vi "Pressure_control_April2018.vi"(7 "Run Sequence":bool, 8 "user sequence, present (s) in, current step in, seq time in":T7, 9 "pressure parameters in":T4={"valve % open"=100.0, "Desired pressure"=0.0, "set Vapor sccm"=0.0, "set Gas sccm"=0.0, "Valve mode"=enum."% Open", "Pressure Mode"=enum."Abs. pressure", "analyte partial pressure"=100.0} caption="Set pressure parameters" {"analyte partial pressure" min=0.0 max=100.0 step=5.0; "set Gas sccm" min=0 max=200 step=5; "set Vapor sccm" min=0 max=200 step=5; "Desired pressure" min=0.0 max=760.0 step=5.0; "valve % open" min=0.0 max=100.0 step=5.0 format="%#_2f"}, 11 "pressure control on?/daq IDs/errors":T3) -> (0 "current step # out, shift register time out, seq button on?":T6, 1 "sequence over? USE THIS TO REINITIALIZE RUN SEQUENCE BUTTON SO PROGRAM ENDS":bool, 2 "save press/RH/gasflow/vaporflow - read valve position/pressure/vaporflow/gasflow":T5, 3 "pressure control on?/daq IDs/errors out":T2, 4 "sequence end date/time string":string, 5 "abs_t, delta_t, abs_p, delta_p":T1)   [LabVIEW 2014]
uses:
  <vilib>/DAQmx/read.llb/DAQmx Read (Analog 1D DBL NChan 1Samp).vi
  <vilib>/DAQmx/write.llb/DAQmx Write (Analog 1D DBL NChan 1Samp).vi
panel:
  # "100%"
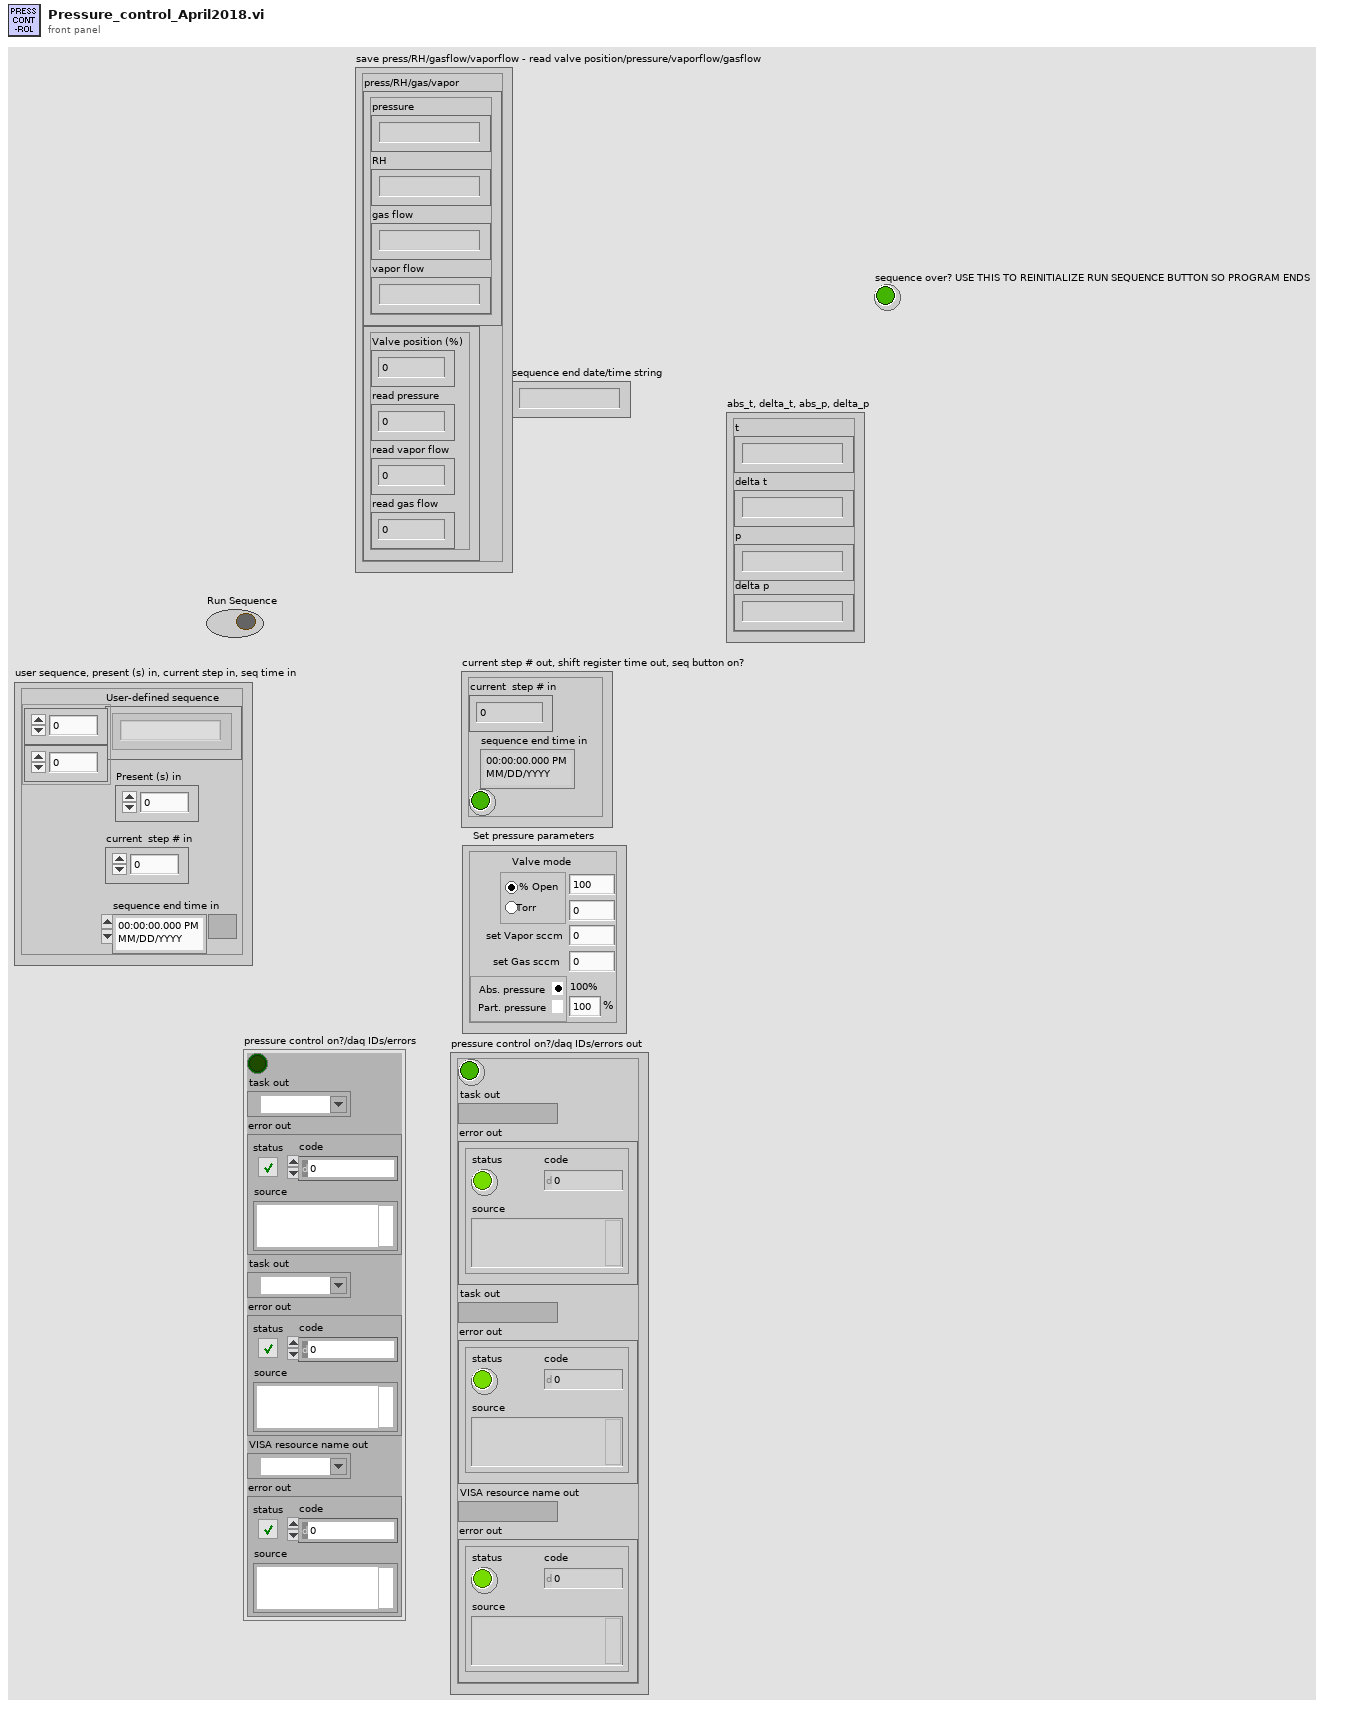
[diagram p1: front panel]
types:
  T1 = cluster{"t":string, "delta t":string, "p":string, "delta p":string}
  T2 = cluster{"Boolean":bool, "task out":refnum<k21>, "error out":errorcluster, "task out":refnum<k21>, "error out":errorcluster, "VISA resource name out":refnum<visa-resource-name>, "error out":errorcluster}
  T3 = cluster{bool, "task out":refnum<k21>, "error out":errorcluster, "task out":refnum<k21>, "error out":errorcluster, "VISA resource name out":refnum<visa-resource-name>, "error out":errorcluster}
  T4 = cluster{"valve % open":dbl, "Desired pressure":dbl, "set Vapor sccm":sgl, "set Gas sccm":sgl, "Valve mode":enum32{"% Open", "Torr "}, "Pressure Mode":enum32{"Abs. pressure", " Part. pressure"}, "analyte partial pressure":dbl}
  T5 = cluster{"press/RH/gas/vapor":cluster{"pressure":string, "RH":string, "gas flow":string, "vapor flow":string}, "Cluster":cluster{"Valve position (%)":dbl, "read pressure":dbl, "read vapor flow":dbl, "read gas flow":dbl}}
  T6 = cluster{"current  step # in":i32, "sequence end time in":timestamp, "Boolean":bool}
  T7 = cluster{"User-defined sequence":string[][], "Present (s) in":dbl, "current  step # in":i32, "sequence end time in":timestamp}
  T8 = cluster{"Elapsed Time (s)":string, "Elapsed Time (s)":string, "String":string, string}
  T9 = cluster{"Valve position (%)":dbl, "pressure":dbl, "vapor flow":dbl, "gas flow":dbl}
  T10 = cluster{"pressure":string, "RH":string, "gas flow":string, "vapor flow":string}
  T11 = cluster{"String":dbl, "String":dbl, "Pressure Control":u32}
  T12 = cluster{"Valve position (%)":dbl, "read pressure":dbl, "read vapor flow":dbl, "read gas flow":dbl}
  T13 = cluster{"Elapsed Time (s)":dbl, "Elapsed Time (s)":dbl, "String":dbl, dbl}
  T14 = cluster{bool, "task out":refnum<k21>, "error out":errorcluster, "task out":refnum<k21>, "error out":errorcluster, "VISA Refnum out":refnum<visa-resource-name>, "error out":errorcluster}
  T15 = cluster{"press/RH/gas/vapor":cluster{"pressure":string, "RH":string, "gas flow":string, "vapor flow":string}, cluster{"Valve position (%)":dbl, "read pressure":dbl, "read vapor flow":dbl, "read gas flow":dbl}}
  T16 = cluster{"current  step # in":i32, "sequence end time in":timestamp, bool}
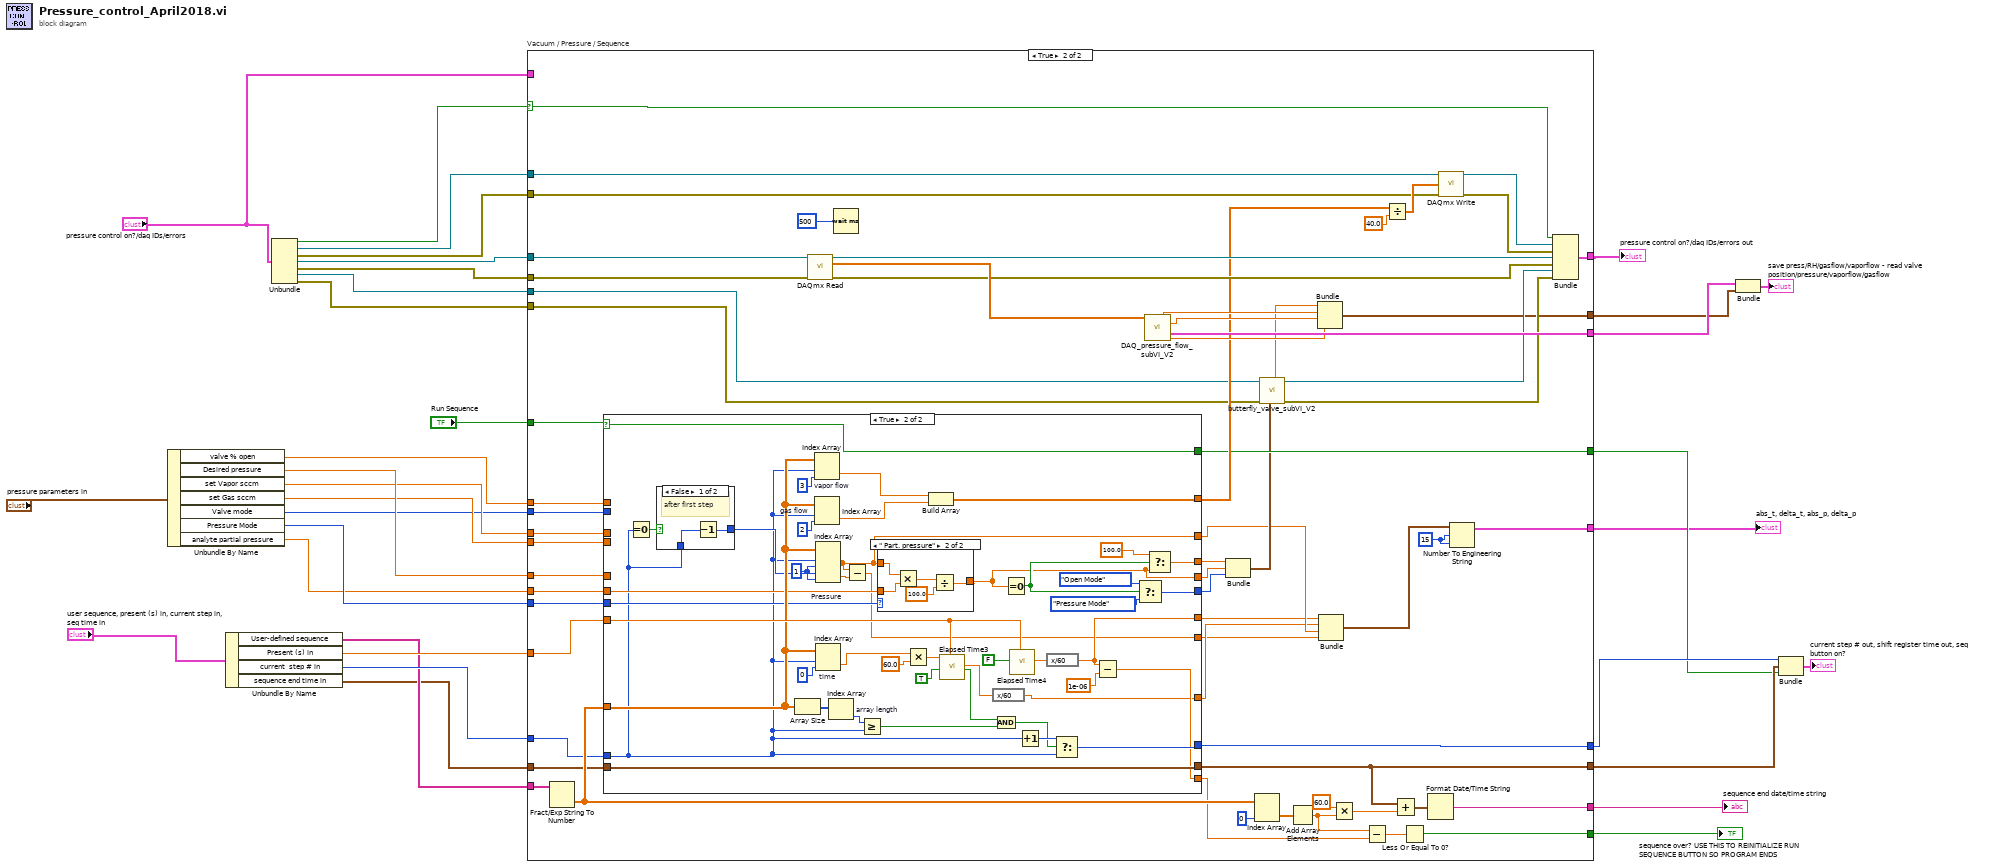
[diagram p0: block diagram]
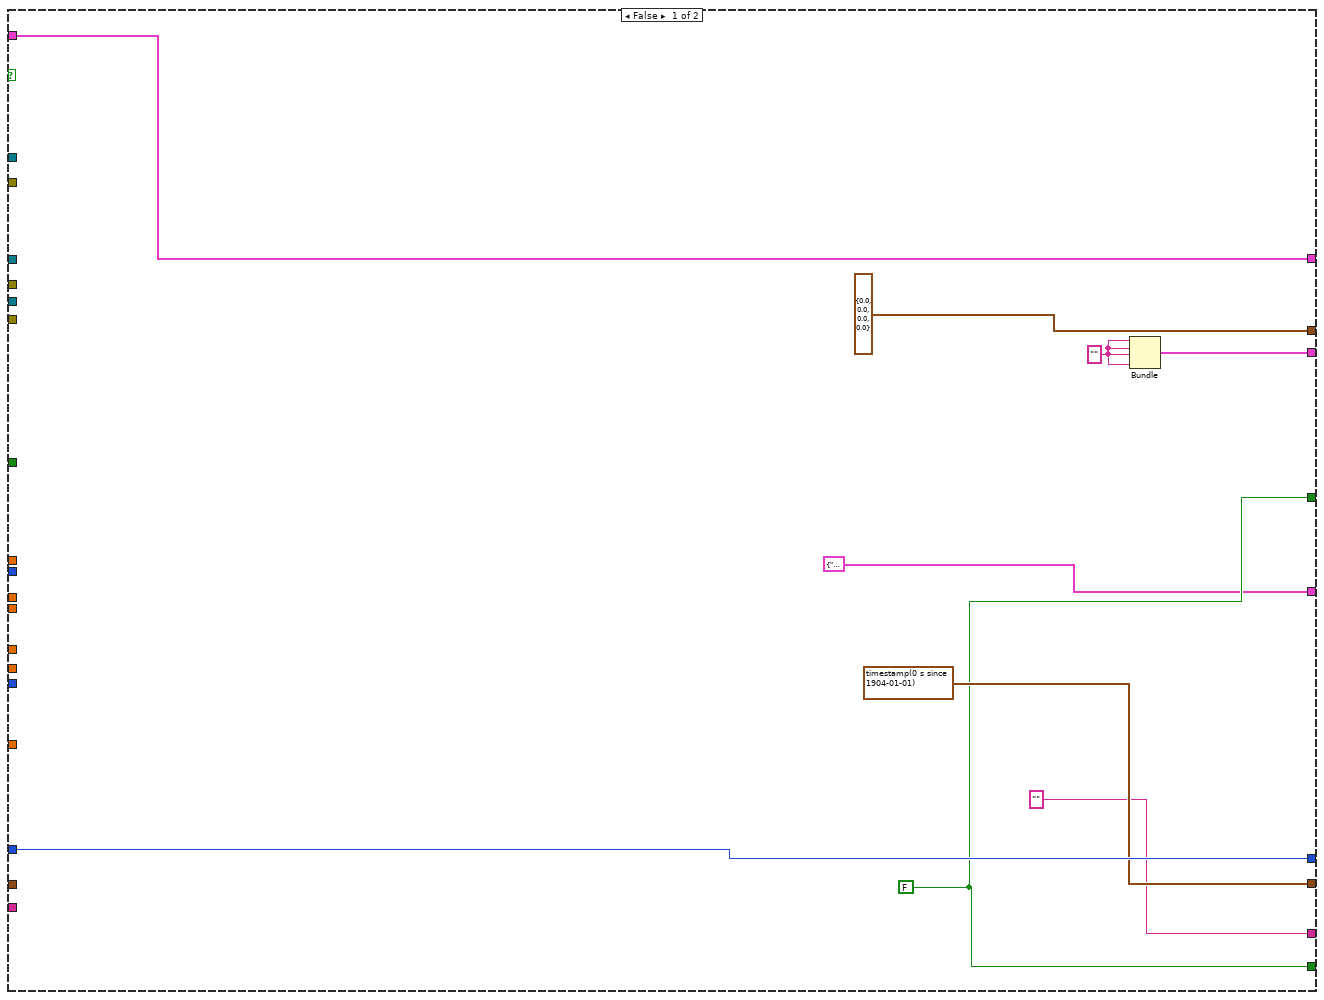
[diagram p2: hidden frame]
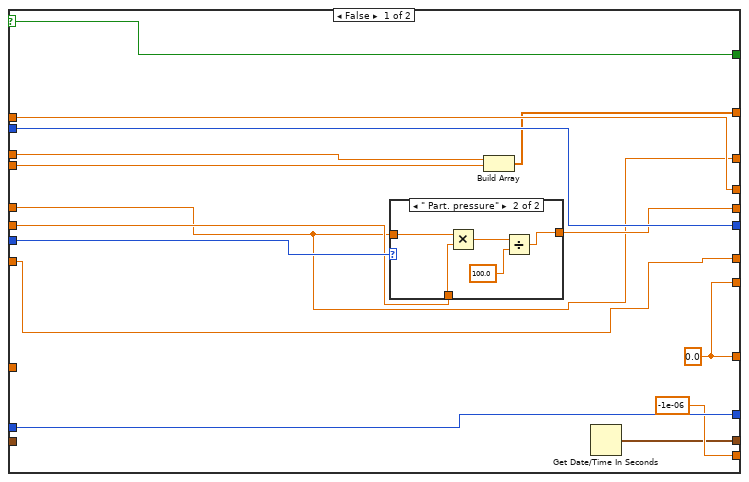
[diagram p3: hidden frame]
diagram:
  n1 = Unbundle By Name("pressure parameters in") -> ("valve % open"=w11:dbl, "Desired pressure"=w15:dbl, "set Vapor sccm"=w13:sgl, "set Gas sccm"=w14:sgl, "Valve mode"=w12:enum32{"% Open", "Torr "}, "Pressure Mode"=w17:enum32{"Abs. pressure", " Part. pressure"}, "analyte partial pressure"=w16:dbl)
  n2 = Unbundle By Name("user sequence, present (s) in, current step in, seq time in") -> ("User-defined sequence"=w27:string[][], "Present (s) in"=w28:dbl, "current  step # in"=w29:i32, "sequence end time in"=w26:timestamp)
  n3 = Unbundle("pressure control on?/daq IDs/errors") -> (w10:bool, "task out"=w9:refnum<k21>, "error out"=w8:errorcluster, "task out"=w7:refnum<k21>, "error out"=w6:errorcluster, "VISA resource name out"=w5:refnum<visa-resource-name>, "error out"=w4:errorcluster)
  n4 = case "Vacuum / Pressure / Sequence" shown="True" w10 {
    selector: w10 -> [_ w50]
    tunnel: w29 -> [w42 w79]
    tunnel: [w42 w59] -> w25
    tunnel: [w37 w77] -> w23
    tunnel: [timestamp(0 s since 1904-01-01) ("seconds since 1Jan1904") w76] -> w24
    tunnel: [w40 w93] -> w21
    tunnel: w27 -> [_ w84]
    tunnel: ["" ("date/time string") w83] -> w33
    tunnel: [T9 {"Valve position (%)"=0.0, "pressure"=0.0, "vapor flow"=0.0, "gas flow"=0.0} w82] -> w20
    tunnel: w28 -> [_ w74]
    tunnel: "Run Sequence" -> [_ w73]
    tunnel: w26 -> [_ w72]
    tunnel: [w37 w71] -> w31
    tunnel: w15 -> [_ w70]
    tunnel: w11 -> [_ w69]
    tunnel: w13 -> [_ w68]
    tunnel: w17 -> [_ w67]
    tunnel: w12 -> [_ w66]
    tunnel: w14 -> [_ w65]
    tunnel: w16 -> [_ w64]
    tunnel: w9 -> [_ w57]
    tunnel: w8 -> [_ w56]
    tunnel: w7 -> [_ w55]
    tunnel: w6 -> [_ w54]
    tunnel: w5 -> [_ w53]
    tunnel: w4 -> [_ w52]
    tunnel: "pressure control on?/daq IDs/errors" -> [w35 _]
    tunnel: [w35 w51] -> w2
    tunnel: [T8 {"Elapsed Time (s)"="", "Elapsed Time (s)"="", "String"="", ""} w45] -> w1
    frame False {
      w37 = FALSE
      w39 = ""
      n5 = Bundle(w39, w39, w39, w39) -> (w40:cluster{string, string, string, string})  [unwired: 1 in]
    }
    frame True {
      w43 = i16 15 ("precision (6)")
      n6 = Fract/Exp String To Number ("user sequence")(string=w84) -> (number=w80:dbl[][])  [unwired: 3 in, 1 out]
      n7 = case "Sequence" shown="True" w73 {
        selector: w73 -> [w116 w154]
        tunnel: w74 -> [w106 w159]
        tunnel: [w119 w160] -> w59
        tunnel: w79 -> [w119 w126]
        tunnel: w65 -> [w114 _]
        tunnel: [w111 w137] -> w63
        tunnel: w80 -> [_ w156]
        tunnel: w66 -> [w118 _]
        tunnel: [w118 w140] -> w62
        tunnel: [-1e-06 w138] -> w75
        tunnel: [w116 w154] -> w77
        tunnel: [w115 w144] -> w58
        tunnel: w69 -> [w115 _]
        tunnel: [w113 w150] -> w78
        tunnel: [w112 w149] -> w76
        tunnel: w72 -> [_ w149]
        tunnel: w70 -> [w107 _]
        tunnel: w64 -> [w108 w148]
        tunnel: w67 -> [w110 w146]
        tunnel: w68 -> [w109 _]
        tunnel: [w107 w128] -> w49
        tunnel: [w106 w135] -> w48
        tunnel: [w105 w133] -> w47
        tunnel: [w105 w127] -> w44
        frame False {
          w105 = 0.0
          n8 = case shown="\" Part. pressure\"" w110 {
            tunnel: [w120 w121] -> w111
            tunnel: w107 -> [w120 w123]
            tunnel: w108 -> [_ w122]
            frame "Abs. pressure", Default {
            }
            frame " Part. pressure" {
              n9 = Multiply(x=w123, y=w122) -> (x*y=w125:dbl)
              n10 = Divide(x=w125, y=100.0 ("Analyte part. press. (%)")) -> (x/y=w121:dbl)
            }
          }
          n11 = Build Array(w109, w114) -> (w113:sgl[])
          n12 = Get Date/Time In Seconds() -> (seconds since 1Jan1904=w112:timestamp)
        }
        frame True {
          w131 = 1 ("disabled index (col)")
          n13 = Equal To 0?(x=w126) -> (x = 0?=w132:bool)
          n14 = case shown="False" w132 {
            tunnel: w126 -> [w171 w172]
            tunnel: [w170 w172] -> w130
            frame False {
              # "after first step"
              n15 = Decrement(x=w171) -> (x-1=w170:i32)
            }
            frame True {
              # "first step"
            }
          }
          n16 = Array Size(array=w156) -> (size(s)=w169:i32[])
          n17 = Index Array "vapor flow"(array=w156, index (row)=w126, index (col)=3 ("disabled index (col)")) -> (element=w152:dbl)
          n18 = Index Array "gas flow"(array=w156, index (row)=w126, index (col)=2 ("disabled index (col)")) -> (element=w151:dbl)
          n19 = Index Array "Pressure"(array=w156, index (row) #1=w126, index (col) #1=w131, index (row) #2=w130, index (col) #2=w131) -> (element #1=w128:dbl, element #2=w129:dbl)
          n20 = Index Array "time"(array=w156, index (row)=w126, index (col)=0) -> (element=w163:dbl)
          n21 = Index Array "array length"(array=w169) -> (element=w157:i32)  [unwired: 1 in]
          n22 = Subtract(x=w128, y=w129) -> (x-y=w127:dbl)
          n23 = Greater Or Equal?(x=w157, y=w126) -> (x >= y?=w166:bool)
          n24 = case shown="\" Part. pressure\"" w146 {
            tunnel: [w173 w174] -> w137
            tunnel: w128 -> [w173 w176]
            tunnel: w148 -> [_ w175]
            frame "Abs. pressure", Default {
            }
            frame " Part. pressure" {
              n25 = Multiply(x=w176, y=w175) -> (x*y=w177:dbl)
              n26 = Divide(x=w177, y=100.0 ("Analyte part. press. (%)")) -> (x/y=w174:dbl)
            }
          }
          n27 = Multiply(x=w163, y=60.0) -> (x*y=w155:dbl)
          n28 = Build Array(w152, w151) -> (w150:dbl[])
          n29 = call "Elapsed Time3"("Time Target (s)"=w155, "Auto Reset"=TRUE, "Set Start Time (s)"=w159) -> ("Elapsed Time (s)"=w134:dbl, "Time has Elapsed"=w147:bool)  [unwired: 9 in, 6 out]
          n30 = expression code="x/60"(w134) -> (w133:dbl)
          n31 = And(x=w147, y=w166) -> (x .and. y?=w153:bool)
          n32 = Equal To 0?(x=w137) -> (x = 0?=w143:bool)
          n33 = call "Elapsed Time4"("Reset"=FALSE, "Set Start Time (s)"=w159) -> ("Elapsed Time (s)"=w136:dbl)  [unwired: 10 in, 7 out]
          n34 = Increment(x=w126) -> (x+1=w161:i32)
          n35 = expression code="x/60"(w136) -> (w135:dbl)
          n36 = Select(t=w161, s=w153, f=w126) -> (s? t:f=w160:i32)
          n37 = Subtract(x=w135, y=1e-06) -> (x-y=w138:dbl)
          n38 = Select(t=enum32{"Open Mode", "Pressure Mode"}."Open Mode" ("Pressure Control"), s=w143, f=enum32{"Open Mode", "Pressure Mode"}."Pressure Mode" ("Pressure Control")) -> (s? t:f=w140:enum32{"Open Mode", "Pressure Mode"})
          n39 = Select(t=100.0 ("valve % open 2"), s=w143, f=w137) -> (s? t:f=w144:dbl)
        }
      }
      n40 = call-poly <vilib>:"DAQmx Read.vi"("task/channels in"=w55, "error in"=w54) -> ("task out"=w90:refnum<k21>, "data"=w103:dbl[], "error out"=w89:errorcluster)  [unwired: 11 in]
      n41 = Wait (ms)(milliseconds to wait=u32 500) -> ()  [unwired: 1 out]
      n42 = call "DAQ_pressure_flow_subVI_V2.vi"("vac press"=w103) -> ("read pressure"=w81:dbl, "read vapor flow"=w86:dbl, "press/RH/gas/vapor"=w93:T10, "read gas flow"=w85:dbl)  [unwired: 11 in]
      n43 = Bundle("String"=w58, "String"=w63, "Pressure Control"=w62) -> (w60:T11)  [unwired: 1 in]
      n44 = Index Array(array=w80, index (col)=0 ("disabled index (col)")) -> (element=w100:dbl[])  [unwired: 1 in]
      n45 = call "butterfly_valve_subVI_V2.vi"("% open / desired pressure / pressure mode"=w60, "error in (no error)"=w52, "VISA Refnum in"=w53) -> ("error out"=w87:errorcluster, "VISA Refnum out"=w88:refnum<visa-resource-name>, "Valve position (%)"=w61:dbl)  [unwired: 6 in]
      n46 = Add Array Elements(numeric array=w100) -> (sum=w94:dbl)
      n47 = Bundle("Valve position (%)"=w61, "read pressure"=w81, "read vapor flow"=w86, "read gas flow"=w85) -> (w82:T12)  [unwired: 1 in]
      n48 = Bundle("Elapsed Time (s)"=w48, "Elapsed Time (s)"=w47, "String"=w49, w44) -> (w46:T13)  [unwired: 1 in]
      n49 = Multiply(x=60.0 ("y"), y=w94) -> (x*y=w96:dbl)
      n50 = Subtract(x=w94, y=w75) -> (x-y=w98:dbl)
      n51 = Divide(x=w78, y=40.0 ("Waveform")) -> (x/y=w102:dbl[])
      n52 = Add(x=w76, y=w96) -> (x+y=w95:timestamp)
      n53 = Less Or Equal To 0?(x=w98) -> (x <= 0?=w71:bool)
      n54 = Format Date/Time String(seconds (now)=w95) -> (date/time string=w83:string)  [unwired: 2 in]
      n55 = call-poly <vilib>:"DAQmx Write.vi"("task/channels in"=w57, "data"=w102, "error in"=w56) -> ("task out"=w92:refnum<k21>, "error out"=w91:errorcluster)  [unwired: 10 in, 1 out]
      n56 = Number To Engineering String(2:w43, 3:w43, 4:w46) -> (0:w45:T8)  [unwired: 1 in]
      n57 = Bundle(w50, "task out"=w92, "error out"=w91, "task out"=w90, "error out"=w89, "VISA Refnum out"=w88, "error out"=w87) -> (w51:T14)  [unwired: 1 in]
    }
  }
  "sequence end date/time string" <- w33
  "sequence over? USE THIS TO REINITIALIZE RUN SEQUENCE BUTTON SO PROGRAM ENDS" <- w31
  "pressure control on?/daq IDs/errors out" <- w2
  "abs_t, delta_t, abs_p, delta_p" <- w1
  n58 = Bundle("press/RH/gas/vapor"=w21, w20) -> (→"save press/RH/gasflow/vaporflow - read valve position/pressure/vaporflow/gasflow":T15)  [unwired: 1 in]
  n59 = Bundle("current  step # in"=w25, "sequence end time in"=w24, w23) -> (→"current step # out, shift register time out, seq button on?":T16)  [unwired: 1 in]
